vi "AFscanFirstPeak.vi"(6 "StopAfterMaxFrac":dbl=0.9 format="%#_13g", 7 "ScanRange":dbl=1.0, 8 "error in (no error)":errorcluster, 9 "ImageIn":T1, 10 "SessionIn":T2 caption="Session In", 11 "controller in":refnum<k24>) -> (0 "error out":errorcluster, 1 "Image Out":T1, 2 "Session Out":T2, 3 "controller out":refnum<k24>, 4 "MaxVal":dbl, 5 "BestZ":dbl)   [LabVIEW 2021]
uses:
  C:/Users/TTUHEP/Documents/LabVIEW/Other Models/2010/Bin/Aerotech.A3200.dll
  Other Models/2010/Bin/Aerotech.A3200.dll
  <vilib>/userDefined/High Color/IMAQdx.ctl
  <vilib>/vision/Image Controls.llb/IMAQ Image.ctl
  GlobalVariables.vi
  Other Models/2010/Motion/AbortSingle.vi
  <vilib>/vision/NI_Vision_Development_Module.lvlib
  <vilib>/vision/driver/NI_Vision_Acquisition_Software.lvlib
panel:
  out "Array 2":sgl[](array[numeric])
  out "Array":dbl[](array[numeric])
  out "XY Graph":T3(graph)
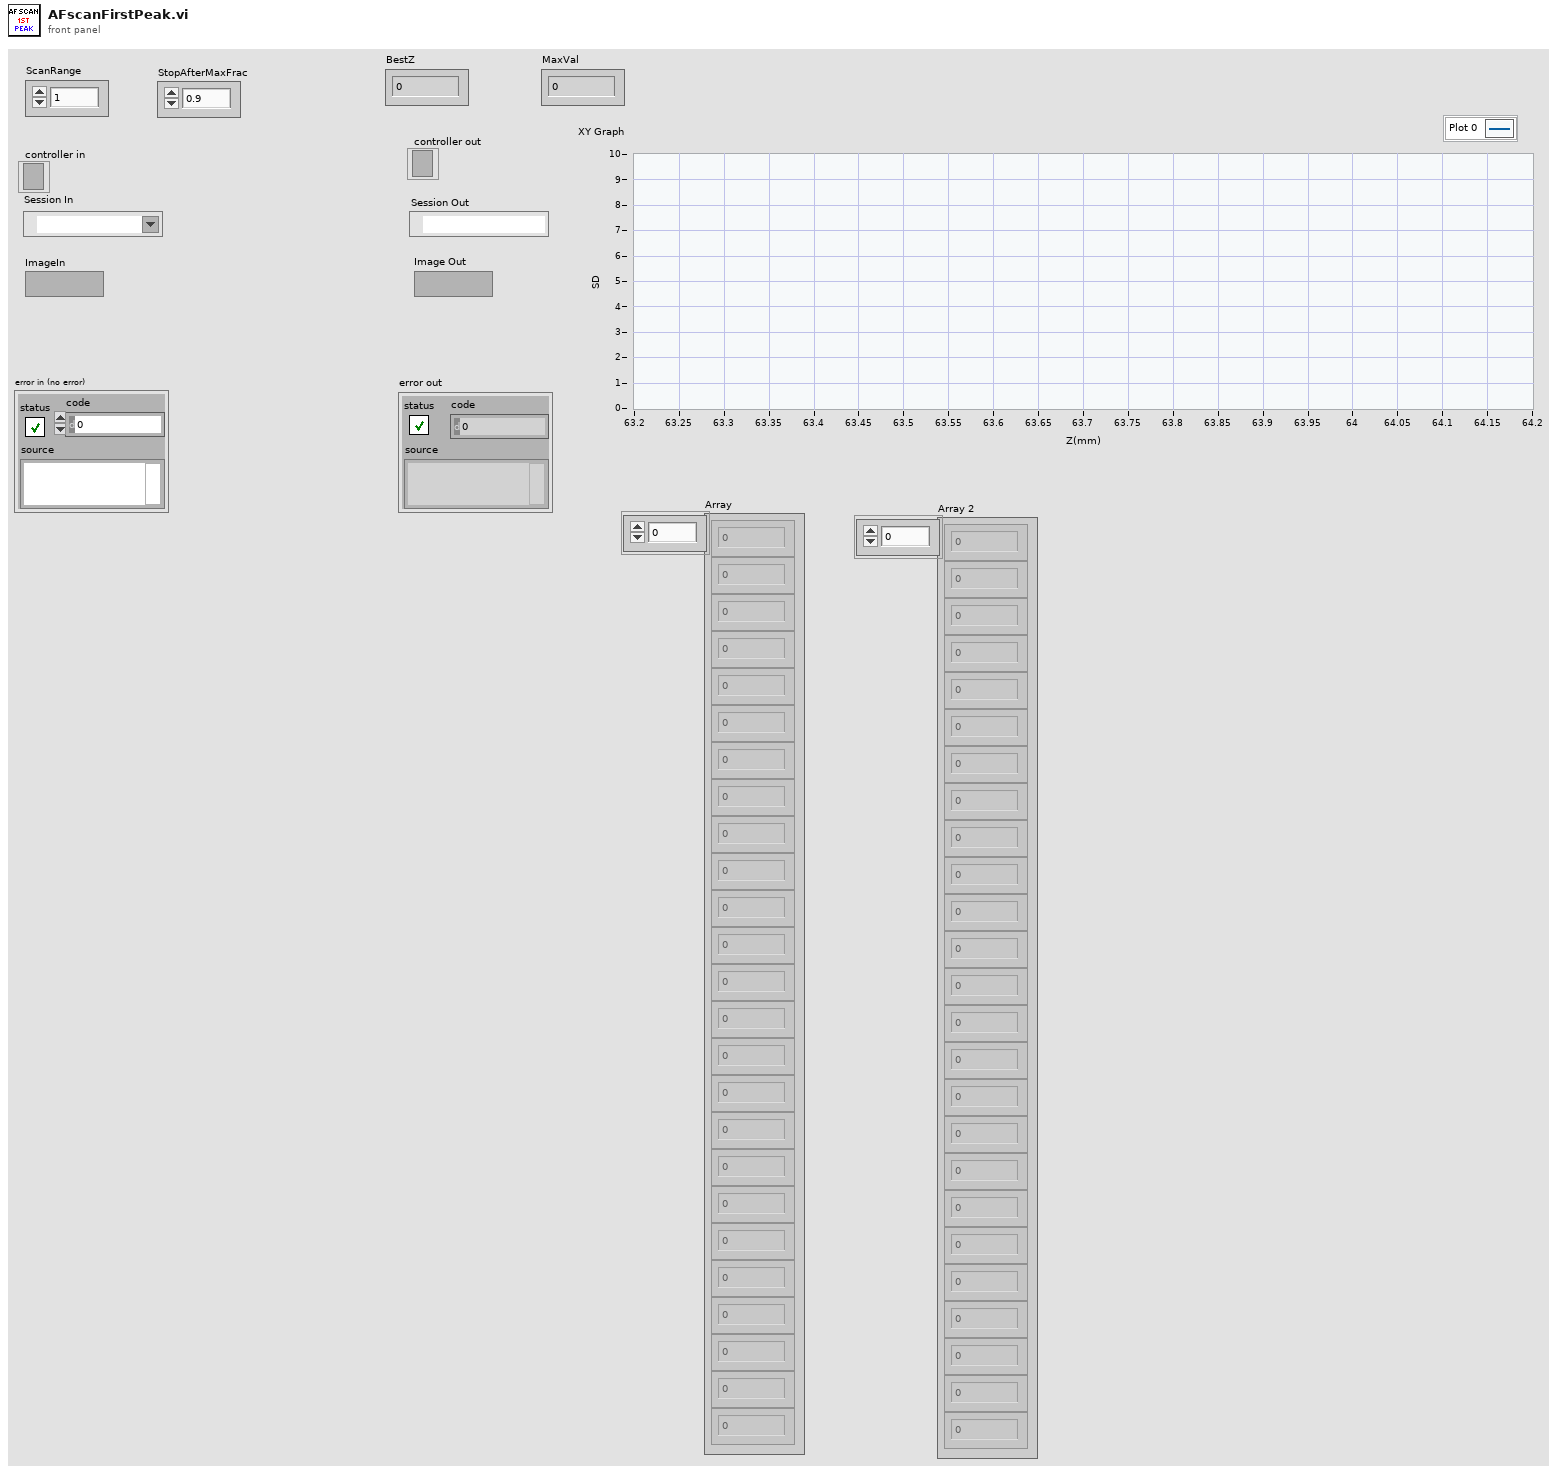
[diagram p1: front panel]
types:
  T1 = typedef "IMAQ Image.ctl" = refnum<image>
  T2 = typedef "IMAQdx.ctl" = refnum<k21>
  T3 = cluster{"Position Z":dbl, "Standard  Deviation":sgl}[]
  T4 = enum32{"Differentiation", "Gradient", "Prewitt", "Roberts", "Sigma", "Sobel"}
  T5 = typedef "Image Type" = u32
  T6 = cluster{"Position Z":dbl, "Standard  Deviation":sgl}
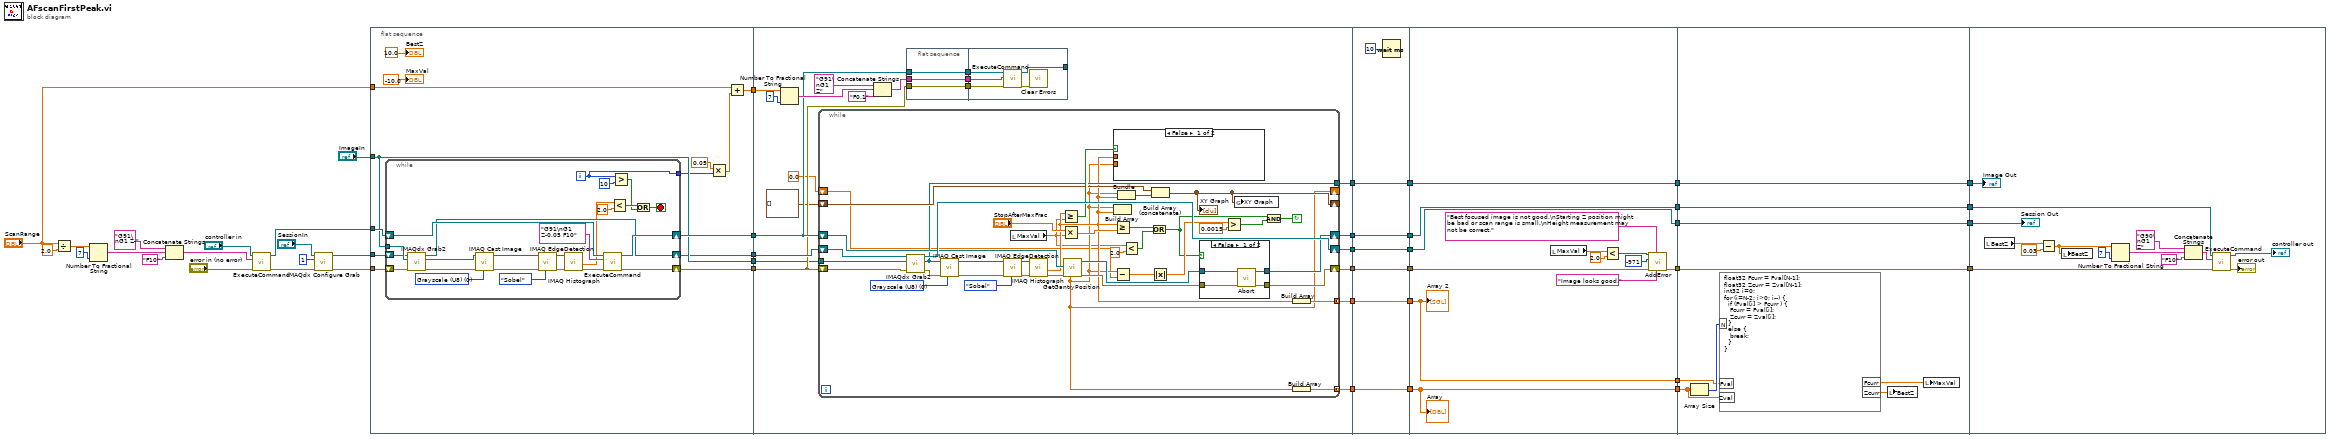
[diagram p0: block diagram]
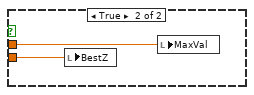
[diagram p3: hidden frame]
diagram:
  n1 = Divide(x="ScanRange", y=2.0) -> (x/y=w28:dbl)
  n2 = Number To Fractional String(number=w28, precision (6)=i16 7) -> (F-format string=w27:string)  [unwired: 2 in]
  n3 = Concatenate Strings("G91\nG1 Z-", w27, "F10" ("string")) -> (w26:string)
  n4 = call "ExecuteCommand.vi"("error in (no error)"="error in (no error)", "Command Code"=w26, "controller in"="controller in") -> ("error out"=w23:errorcluster, "controller out"=w35:refnum<k24>)  [unwired: 6 in, 1 out]
  n5 = call <vilib>:"IMAQdx Configure Grab.vi"("error in"=w23, "Number of Buffers"=u32 1, "Session In"="SessionIn") -> ("error out"=w22:errorcluster, "Session Out"=w34:T2)  [unwired: 7 in]
  n6 = flat-sequence {
    tunnel: w34 -> [w51]
    tunnel: w22 -> [w54]
    tunnel: "ImageIn" -> [w52]
    tunnel: "ScanRange" -> [w47]
    tunnel: w35 -> [w56]
    tunnel: [w55] -> w44
    tunnel: [w45] -> w43
    tunnel: [w52] -> w42
    tunnel: [w53] -> w41
    tunnel: [w50] -> w40
    tunnel: w44 -> [w94]
    tunnel: w43 -> [w103]
    tunnel: w42 -> [w86]
    tunnel: w41 -> [w93]
    tunnel: w40 -> [w100]
    tunnel: [w89] -> w39
    tunnel: [w102] -> w38
    tunnel: [w101] -> w37
    tunnel: [w87] -> w19
    tunnel: [w85] -> w14
    tunnel: [w84] -> w13
    tunnel: w39 -> [w165]
    tunnel: [w165] -> w12
    tunnel: w38 -> [w164]
    tunnel: [w164] -> w10
    tunnel: w37 -> [w163]
    tunnel: [w163] -> w8
    tunnel: [w161] -> w6
    tunnel: w19 -> [w161]
    tunnel: [w160] -> w4
    tunnel: w14 -> [w160]
    tunnel: [w159] -> w2
    tunnel: w13 -> [w159]
    tunnel: w12 -> [w178]
    tunnel: [w178] -> w11
    tunnel: w10 -> [w177]
    tunnel: [w177] -> w9
    tunnel: w8 -> [w169]
    tunnel: [w167] -> w7
    tunnel: w6 -> [w176]
    tunnel: [w176] -> w5
    tunnel: w4 -> [w175]
    tunnel: [w175] -> w3
    tunnel: w2 -> [w174]
    tunnel: [w174] -> w1
    tunnel: w11 -> [w187]
    tunnel: [w187] -> w18
    tunnel: w9 -> [w186]
    tunnel: [w186] -> w17
    tunnel: w7 -> [w185]
    tunnel: [w185] -> w16
    tunnel: w5 -> [w184]
    tunnel: [w184] -> w15
    tunnel: w3 -> [w180]
    tunnel: w1 -> [w179]
    tunnel: w18 -> [w201]
    tunnel: w17 -> [w191]
    tunnel: w16 -> [w195]
    tunnel: w15 -> [w189]
    frame #0 {
      n7 = while {
        tunnel: w52 -> [w69]
        shift-right: [w74] -> w55
        shift-left: w56 -> [w75]
        shift-right: [w71] -> w53
        shift-left: w54 -> [w72]
        shift-right: [w67] -> w50
        shift-left: w51 -> [w68]
        tunnel: [w59] -> w48
        i -> [w59]
        stop <- w60 stop-if-true
        w81 = T5 0 items=["Grayscale (U8)", "Grayscale (I16)", "Grayscale (SGL)", "Complex (CSG)", "RGB (U32)", "HSL (U32)", "RGB (U64)", "Grayscale (U16)"] ("Image Type")
        n8 = call <vilib>:"IMAQdx Grab2.vi"("error in"=w72, "Image In"=w69, "Session In"=w68) -> ("error out"=w78:errorcluster, "Image Out"=w77:T1, "Session Out"=w67:T2)  [unwired: 5 in, 1 out]
        n9 = call "IMAQ Cast Image"("Image Type"=w81, "error in (no error)"=w78, "Image Src"=w77) -> ("error out"=w82:errorcluster, "Image Dst Out"=w76:T1)  [unwired: 7 in]
        n10 = call "IMAQ EdgeDetection"("Method"=T4."Sobel", "error in (no error)"=w82, "Image Src"=w76) -> ("error out"=w80:errorcluster, "Image Dst Out"=w66:T1)  [unwired: 7 in]
        n11 = call "IMAQ Histograph"("error in (no error)"=w80, "Image"=w66) -> ("error out"=w73:errorcluster, "Standard  Deviation"=w65:sgl)  [unwired: 6 in, 2 out]
        n12 = call "ExecuteCommand.vi"("error in (no error)"=w73, "Command Code"="G91\nG1 Z-0.05 F10", "controller in"=w75) -> ("error out"=w71:errorcluster, "controller out"=w74:refnum<k24>)  [unwired: 6 in, 1 out]
        n13 = Less?(x=w65, y=sgl 2.0) -> (x < y?=w62:bool)
        n14 = Greater?(x=w59, y=10) -> (0:w61:bool)
        n15 = Or(x=w62, y=w61) -> (x .or. y?=w60:bool)
      }
      n16 = Multiply(x=0.05, y=w48) -> (x*y=w46:dbl)
      n17 = Add(x=w47, y=w46) -> (x+y=w45:dbl)
      "BestZ" <- 10.0 ("BestZ")
      "MaxVal" <- -10.0 ("MaxVal")
    }
    frame #1 {
      n18 = Number To Fractional String(number=w103, precision (6)=i16 7) -> (F-format string=w97:string)  [unwired: 2 in]
      n19 = while {
        tunnel: w86 -> [w142]
        shift-right: [w141] -> w102
        shift-left: w100 -> [w120]
        shift-right: [w128] -> w89
        shift-left: w94 -> [w134]
        shift-right: [w126] -> w101
        shift-left: w93 -> [w131]
        shift-right: [w123] -> _
        shift-left: T3 [] -> [w124]
        tunnel: [w119] -> w87
        tunnel: [w117] -> w84 mode=concatenating
        tunnel: [w116] -> w85 mode=concatenating
        shift-right: [w115] -> _
        shift-left: 0.0 -> [w114]
        stop <- w109 continue-if-true
        w138 = T5 0 items=["Grayscale (U8)", "Grayscale (I16)", "Grayscale (SGL)", "Complex (CSG)", "RGB (U32)", "HSL (U32)", "RGB (U64)", "Grayscale (U16)"] ("Image Type")
        n20 = call <vilib>:"IMAQdx Grab2.vi"("error in"=w131, "Image In"=w142, "Session In"=w120) -> ("error out"=w130:errorcluster, "Image Out"=w119:T1, "Session Out"=w141:T2)  [unwired: 5 in, 1 out]
        n21 = call "IMAQ Cast Image"("Image Type"=w138, "error in (no error)"=w130, "Image Src"=w119) -> ("error out"=w140:errorcluster, "Image Dst Out"=w139:T1)  [unwired: 7 in]
        n22 = call "IMAQ EdgeDetection"("Method"=T4."Sobel", "error in (no error)"=w140, "Image Src"=w139) -> ("error out"=w137:errorcluster, "Image Dst Out"=w136:T1)  [unwired: 7 in]
        n23 = local read "MaxVal"() -> (w104:dbl)
        n24 = call "IMAQ Histograph"("error in (no error)"=w137, "Image"=w136) -> ("error out"=w133:errorcluster, "Standard  Deviation"=w118:sgl)  [unwired: 6 in, 2 out]
        n25 = Greater Or Equal?(x=w118, y=w104) -> (x >= y?=w132:bool)
        n26 = Multiply(x="StopAfterMaxFrac", y=w104) -> (x*y=w121:dbl)
        n27 = call "GetGantryPosition.vi"("error in (no error)"=w133, "Controller In"=w134) -> ("error out"=w127:errorcluster, "controller out"=w129:refnum<k24>, "Position Z"=w115:dbl)  [unwired: 3 in, 4 out]
        n28 = case shown="False" w132 {
          tunnel: w118 -> [_ w150]
          tunnel: w115 -> [_ w149]
          frame False {
          }
          frame True {
            n29 = local write "BestZ"(w149) -> ()
            n30 = local write "MaxVal"(w150) -> ()
          }
        }
        n31 = Build Array(w115, w118) -> ()  [unwired: 1 out]
        n32 = Greater Or Equal?(x=w118, y=w121) -> (x >= y?=w105:bool)
        n33 = Subtract(x=w115, y=w114) -> (x-y=w113:dbl)
        n34 = Bundle("Position Z"=w115, "Standard  Deviation"=w118) -> (w125:T6)  [unwired: 1 in]
        n35 = Less?(x=w104, y=2.0) -> (x < y?=w108:bool)
        n36 = Or(x=w105, y=w108) -> (x .or. y?=w106:bool)
        n37 = Build Array (concatenate)(w124, w125) -> (w123:T3)
        "XY Graph" <- w123
        n38 = Absolute Value(x=w113) -> (abs(x)=w112:dbl)
        n39 = case shown="False" w106 {
          tunnel: w129 -> [w146 w148]
          tunnel: [w145 w148] -> w128
          tunnel: w127 -> [w144 w147]
          tunnel: [w143 w147] -> w126
          frame False {
            n40 = call-poly "Abort.vi"("error in (no error)"=w144, "controller in"=w146) -> ("error out"=w143:errorcluster, "controller out"=w145:refnum<k24>)  [unwired: 8 in]
          }
          frame True {
          }
        }
        n41 = Greater?(x=w112, y=0.0015) -> (0:w110:bool)
        n42 = global write "GlobalVariables.vi" "XY Graph"(w123) -> ()
        n43 = And(x=w106, y=w110) -> (x .and. y?=w109:bool)
        n44 = Build Array(w118) -> (w117:sgl[])
        n45 = Build Array(w115) -> (w116:dbl[])
      }
      n46 = Concatenate Strings("G91\nG1 Z", w97, "F0.1" ("string")) -> (w96:string)
      n47 = flat-sequence {
        tunnel: w93 -> [w151]
        tunnel: w96 -> [w152]
        tunnel: w94 -> [w153]
        tunnel: [w153] -> w92
        tunnel: [w152] -> w91
        tunnel: [w151] -> w90
        tunnel: w92 -> [w158]
        tunnel: w91 -> [w157]
        tunnel: w90 -> [w156]
        tunnel: [w155] -> _
        frame #0 {
        }
        frame #1 {
          n48 = call "ExecuteCommand.vi"("error in (no error)"=w156, "Command Code"=w157, "controller in"=w158) -> ("error out"=w154:errorcluster, "controller out"=w155:refnum<k24>)  [unwired: 6 in, 1 out]
          n49 = call <vilib>:"Clear Errors.vi"("error in (no error)"=w154) -> ()  [unwired: 5 in, 2 out]
        }
      }
    }
    frame #2 {
      n50 = Wait (ms)(milliseconds to wait=u32 10) -> ()  [unwired: 1 out]
    }
    frame #3 {
      n51 = local read "MaxVal"() -> (w173:dbl)
      n52 = Less?(x=w173, y=2.0) -> (x < y?=w170:bool)
      n53 = call "AddError.vi"("NoErrorMessage"="Image looks good.", "ErrorMessage"="Best focused image is not good.\nStarting Z position might be bad or scan range is small.\nHeight measurement may not be correct." ("message"), "error in"=w169, "code"=-971, "Error?"=w170) -> ("Error out"=w167:errorcluster)  [unwired: 6 in]
      "Array" <- w175
      "Array 2" <- w174
    }
    frame #4 {
      n54 = Array Size(array=w180) -> (size(s)=w183:i32)
      n55 = formula code="float32 Fcurr = Fval[N-1];\nfloat32 Zcurr = Zval[N-1];\nint32 i=0;\nfor (i=N-2; i>0; i--) {\n  if (Fval[i] > Fcurr ) {\n   Fcurr = Fval[i];\n   Zcurr = Zval[i];\n  }\n  else {\n   break;\n  }\n}"("N"=w183, "Fval"=w179, "Zval"=w180) -> ("Fcurr"=w182:sgl, "Zcurr"=w181:sgl)
      n56 = local write "BestZ"(w181) -> ()
      n57 = local write "MaxVal"(w182) -> ()
    }
    frame #5 {
      n58 = local read "BestZ"() -> (w194:dbl)
      n59 = Subtract(x=w194, y=0.03) -> (x-y=w192:dbl)
      n60 = local write "BestZ"(w192) -> ()
      n61 = Number To Fractional String(number=w192, precision (6)=i16 7) -> (F-format string=w197:string)  [unwired: 2 in]
      n62 = Concatenate Strings("G90\nG1 Z", w197, "F10" ("string")) -> (w196:string)
      n63 = call "ExecuteCommand.vi"("error in (no error)"=w195, "Command Code"=w196, "controller in"=w201) -> ("error out"=→"error out":errorcluster, "controller out"=→"controller out":refnum<k24>)  [unwired: 6 in, 1 out]
      "Session Out" <- w191
      "Image Out" <- w189
    }
  }
